vi "Read Transition Time Settings.vi"(0 "VISA resource name":refnum<visa-resource-name>, 11 "error in (no error)":errorcluster) -> (3 "Delay Time (s)":dbl, 4 "VISA resource name out":refnum<visa-resource-name>, 6 "Ramp Up Time (s)":dbl, 8 "Ramp Down Time (s)":dbl, 10 "Dwell Time (s)":dbl, 15 "error out":errorcluster)   [LabVIEW 2016, in "APT 300XAC Series.lvlib"]
doc: "Reads the ramp up time, ramp down time, dwell time and delay time configured in the power source instrument.\n\nNote : Should be used in program mode only."
uses:
  APT 300XAC Series.lvlib
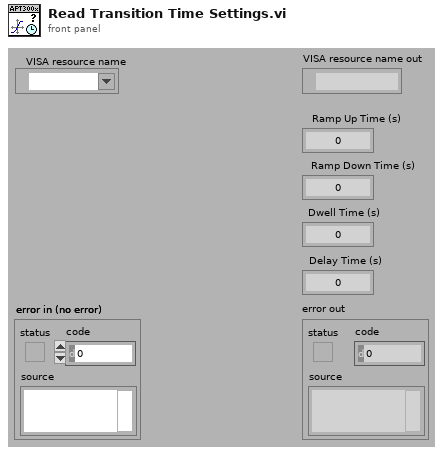
[diagram p1: front panel]
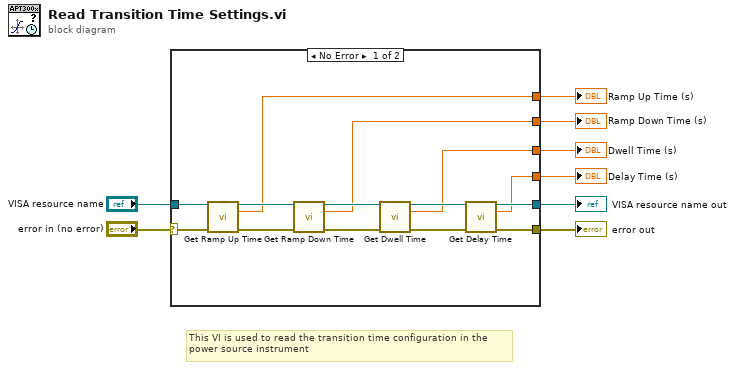
[diagram p0: block diagram]
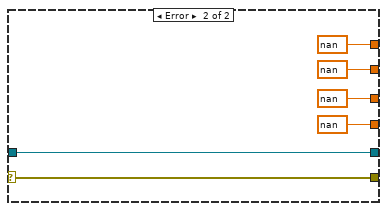
[diagram p2: hidden frame]
diagram:
  # "This VI is used to read the transition time configuration in the\npower source instrument"
  n1 = case shown="No Error" "error in (no error)" {
    selector: "error in (no error)" -> [w21 w27]
    tunnel: [w13 w27] -> w7
    tunnel: [w14 w28] -> w6
    tunnel: "VISA resource name" -> [w22 w28]
    tunnel: [w12 nan ("Delay Time")] -> w4
    tunnel: [w9 nan ("Dwell Time")] -> w3
    tunnel: [w11 nan ("Ramp Down Time")] -> w2
    tunnel: [w10 nan ("Ramp Up Time")] -> w1
    frame No Error {
      n2 = call "Get Ramp Up Time.vi"("VISA resource name"=w22, "error in (no error)"=w21) -> ("VISA resource name out"=w20:refnum<visa-resource-name>, "Ramp Up Time (s)"=w10:dbl, "error out"=w19:errorcluster)  [unwired: 11 in]
      n3 = call "Get Ramp Down Time.vi"("VISA resource name"=w20, "error in (no error)"=w19) -> ("VISA resource name out"=w17:refnum<visa-resource-name>, "Ramp Down Time (s)"=w11:dbl, "error out"=w18:errorcluster)  [unwired: 11 in]
      n4 = call "Get Dwell Time.vi"("VISA resource name"=w17, "error in (no error)"=w18) -> ("VISA resource name out"=w15:refnum<visa-resource-name>, "Dwell Time"=w9:dbl, "error out"=w16:errorcluster)  [unwired: 11 in]
      n5 = call "Get Delay Time.vi"("VISA resource name"=w15, "error in (no error)"=w16) -> ("VISA resource name out"=w14:refnum<visa-resource-name>, "Delay Time (s)"=w12:dbl, "error out"=w13:errorcluster)  [unwired: 11 in]
    }
    frame Error {
    }
  }
  "error out" <- w7
  "VISA resource name out" <- w6
  "Delay Time (s)" <- w4
  "Ramp Down Time (s)" <- w2
  "Dwell Time (s)" <- w3
  "Ramp Up Time (s)" <- w1
